vi "Meas_EIS_Spectra_Polar_v5.vi"(9 "output cluster":T1, 10 "testp":T2={"Start F"=1.0, "Stop F"=10000.0, "# Steps"=50, "Init Z Guess"=1.0, "Device #"=0, "Vdrive (V)"=0.1} caption="Test Parameters" {"Vdrive (V)" min=0.0001 max=10; "Device #" min=0 max=10 step=1; "Init Z Guess" format="%_5f"; "# Steps" min=1 max=1800 step=1; "Stop F" min=0.0010000000474974513 max=2000000.0 step=0.001 format="%#_3f"; "Start F" min=0.0010000000474974513 max=2000000.0 step=0.001 format="%#_3f"}, 11 "Output file refnum":refnum<file>) -> ()   [LabVIEW 2018]
uses:
  AC States cntrl.ctl
panel:
  out "Init Z Guess":sgl
  in  "Tab Control":enum32{"Outputs", "TakeData"}(tab)
  out "XY Graph":cluster{sgl, sgl}[](graph)
  out "IERange":i32
  out "IchRange":i32
  out "VchRange":i32
  out "Index no.":i32=1
  out "Zphz":dbl
  out "Zmod":dbl
  out "Zfreq":dbl
  in  "Control Mode":i32(ring)=1 items=["GstatMode", "PstatMode", "ZRAMode", "FRAMode"]
  out "Data Available":bool
  out "Status":enum16{"Ok", "Retry", "Error"}(ring)
  out "NumPoints":i32
  in  "Freqin":sgl=1000.0 format="%#_3g"
  out "event callback refnum":refnum<k27>
  out "Section":string
  out "ReadZ":refnum<k7>
  out "Pstat":refnum<k7>
  out "Device List":refnum<k7>
  out "Data Acquisition Complete":bool
  in  "GAMRYCOMLib.IGamryReadZ":refnum<k7>
  in  "GAMRYCOMLib.IGamryPstat":refnum<k7>
  in  "GAMRYCOMLib.IGamryDeviceList":refnum<k7>
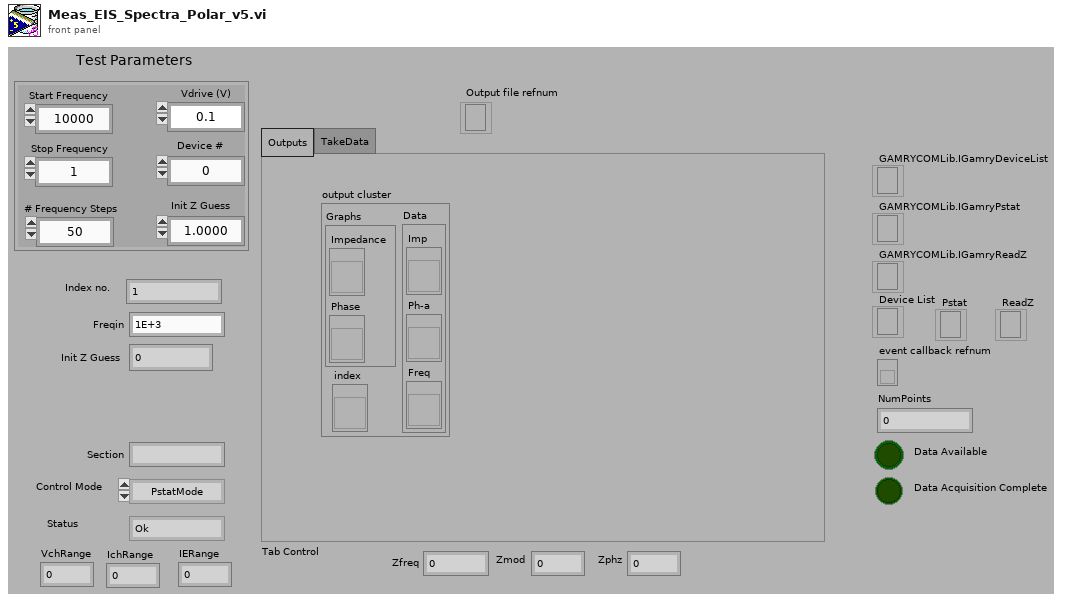
[diagram p1: front panel]
types:
  T1 = cluster{"Data":cluster{"Imp":refnum<vi>, "Ph-a":refnum<vi>, "Freq":refnum<vi>}, "Graphs":cluster{"Impedance":refnum<vi>, "Phase":refnum<vi>}, "index":refnum<vi>}
  T2 = cluster{"Start F":dbl, "Stop F":dbl, "# Steps":u32, "Init Z Guess":sgl, "Device #":i16, "Vdrive (V)":sgl}
  T3 = typedef "AC States cntrl.ctl" = enum16{"Initialize Variables", "Initialize Pstat", "Initialize Dtaq", "Settings", "Frequency calc", "Set Cycle Limits", "Take Data", "Read Z Measure", "Cleanup", "Stop"}
  T4 = cluster{"Imp":refnum<vi>, "Ph-a":refnum<vi>, "Freq":refnum<vi>}
  T5 = cluster{"Impedance":refnum<vi>, "Phase":refnum<vi>}
  T6 = cluster{"Data Acquisition Complete":refnum<vi>, "Status":refnum<vi>}
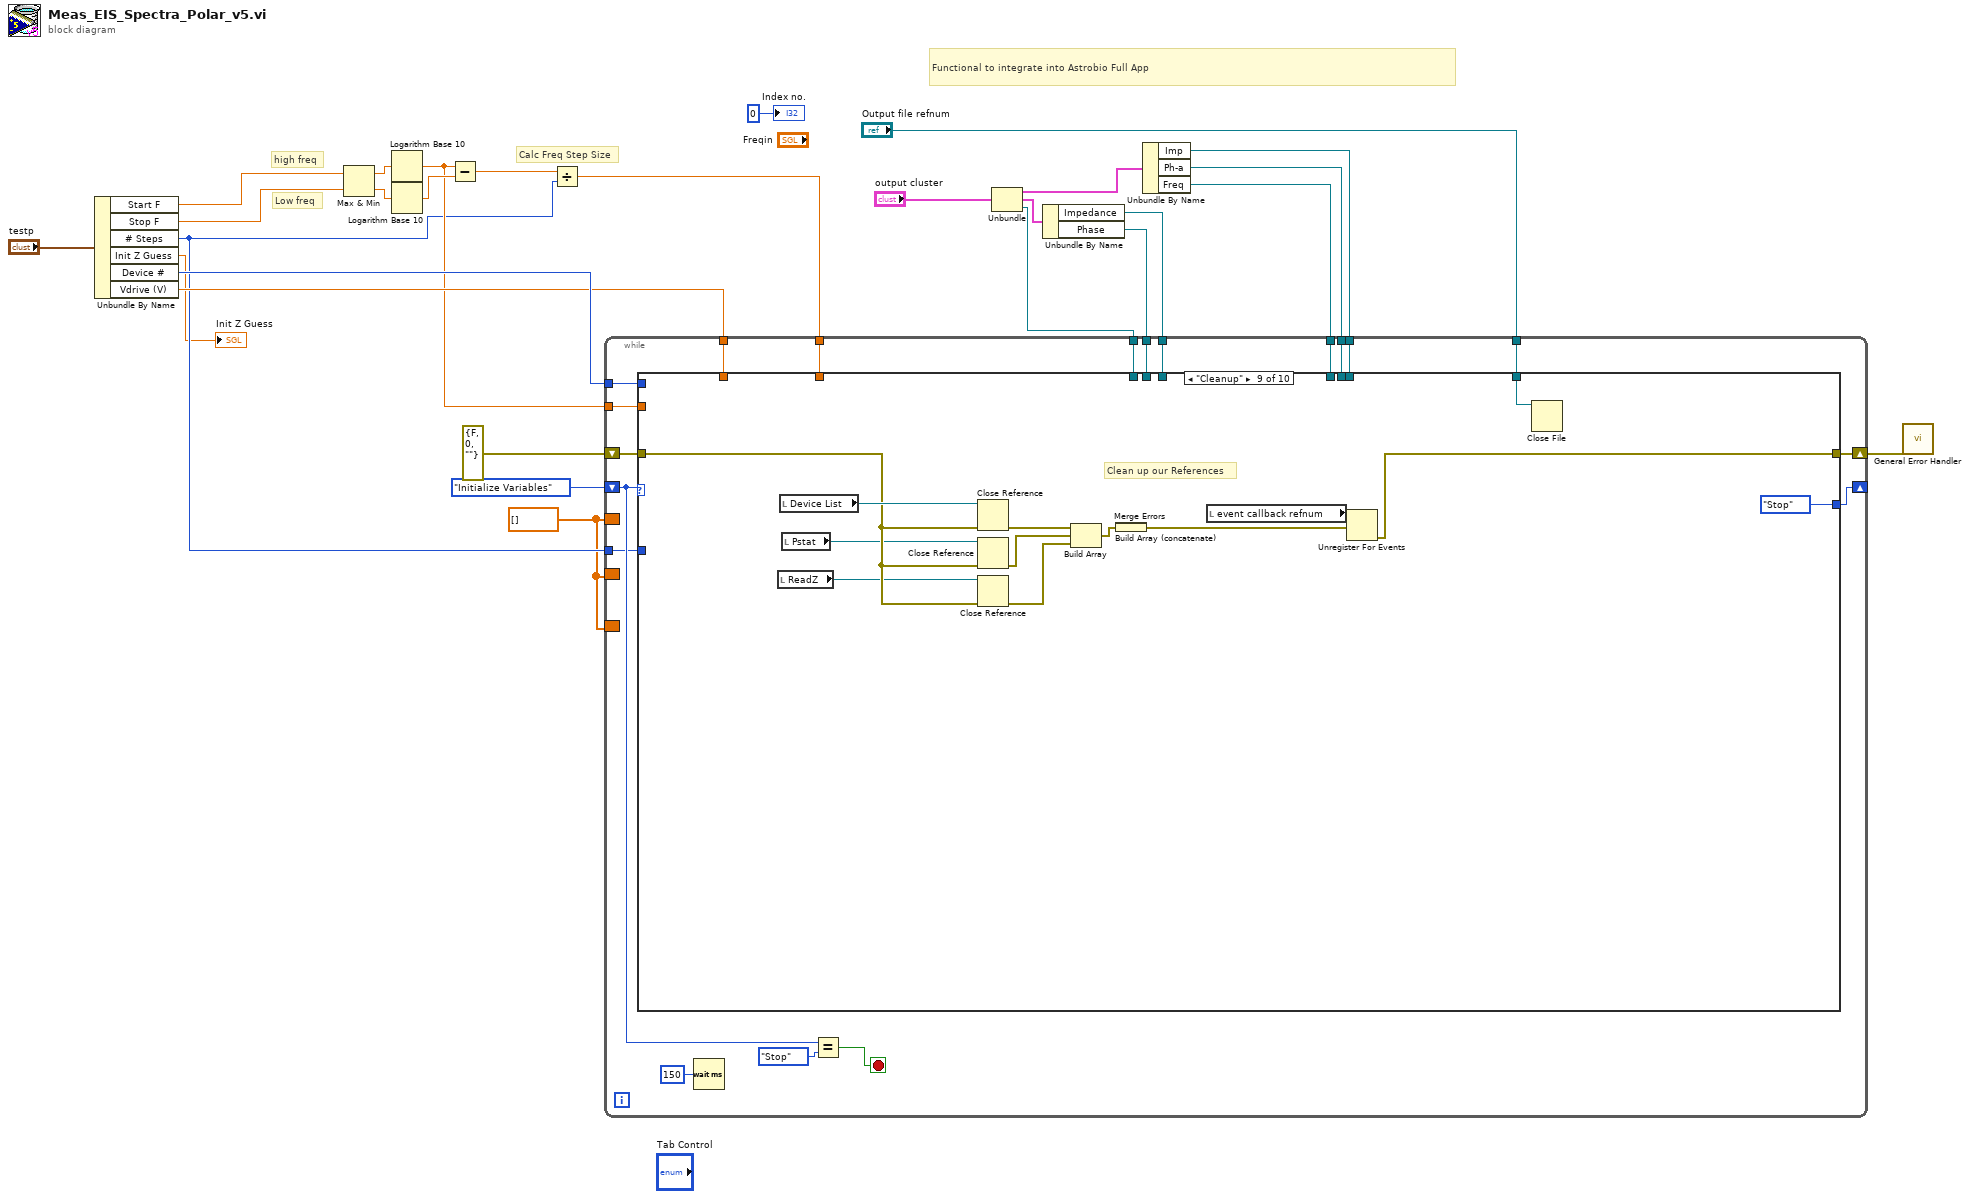
[diagram p0: block diagram]
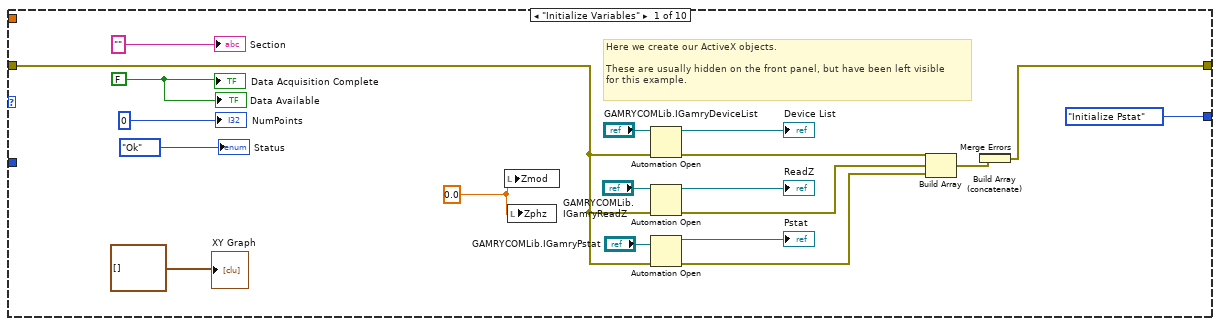
[diagram p2: hidden frame]
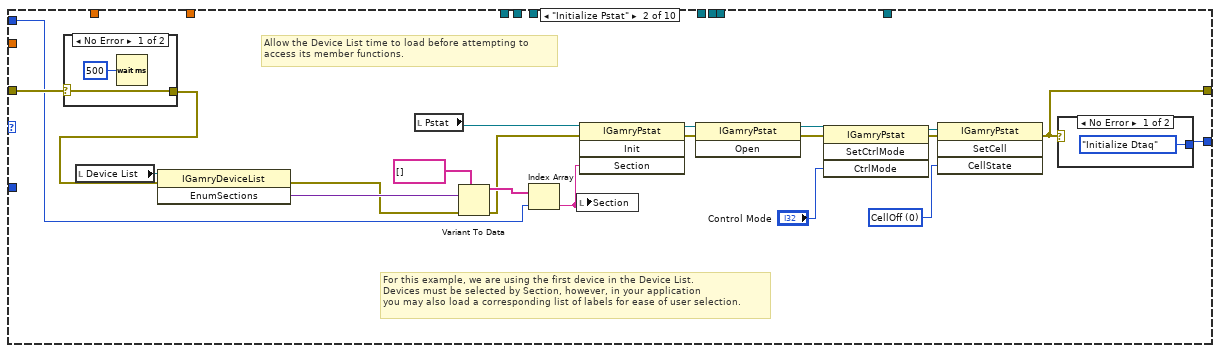
[diagram p3: hidden frame]
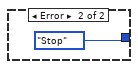
[diagram p5: hidden frame]
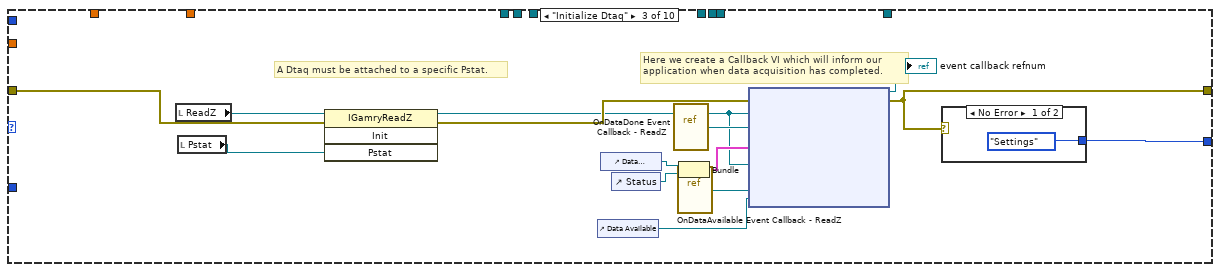
[diagram p6: hidden frame]
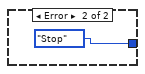
[diagram p7: hidden frame]
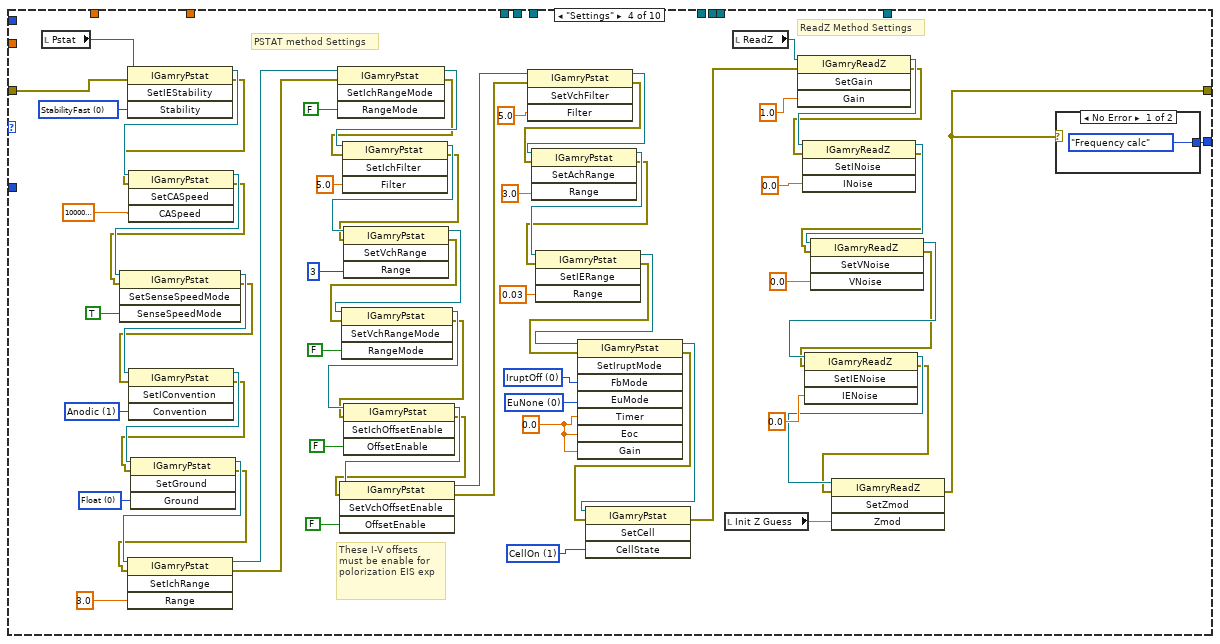
[diagram p8: hidden frame]
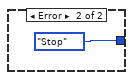
[diagram p9: hidden frame]
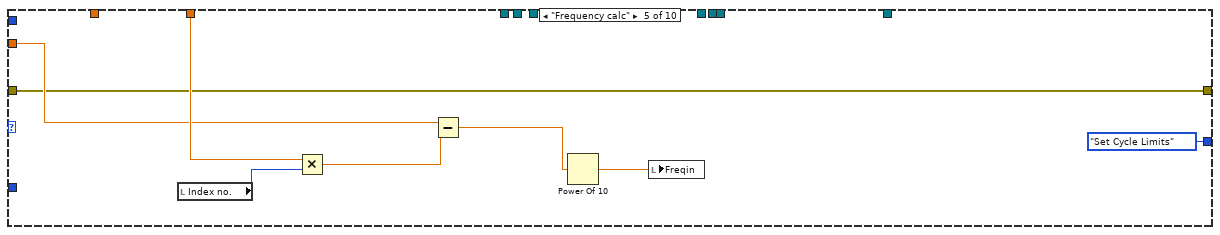
[diagram p10: hidden frame]
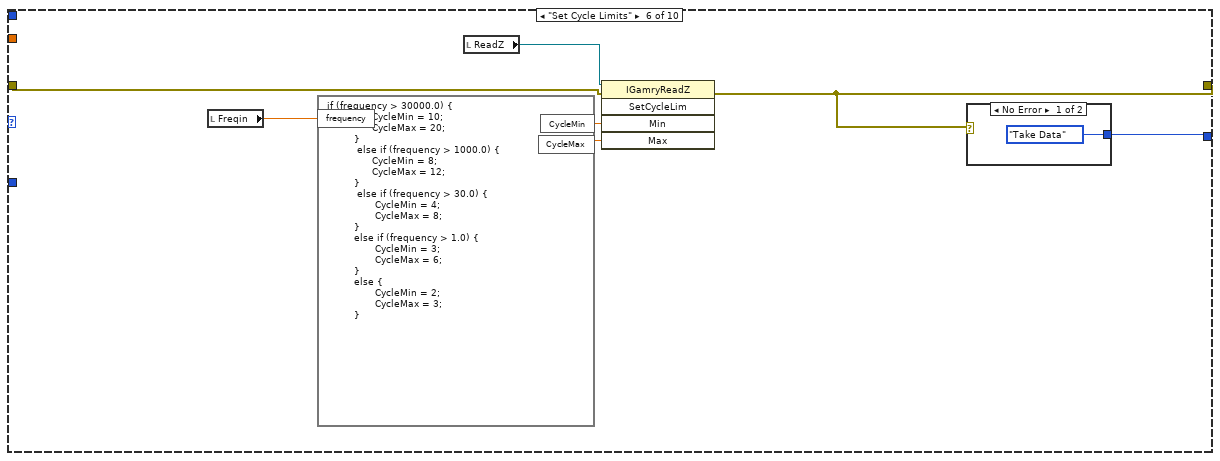
[diagram p11: hidden frame]
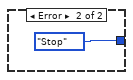
[diagram p12: hidden frame]
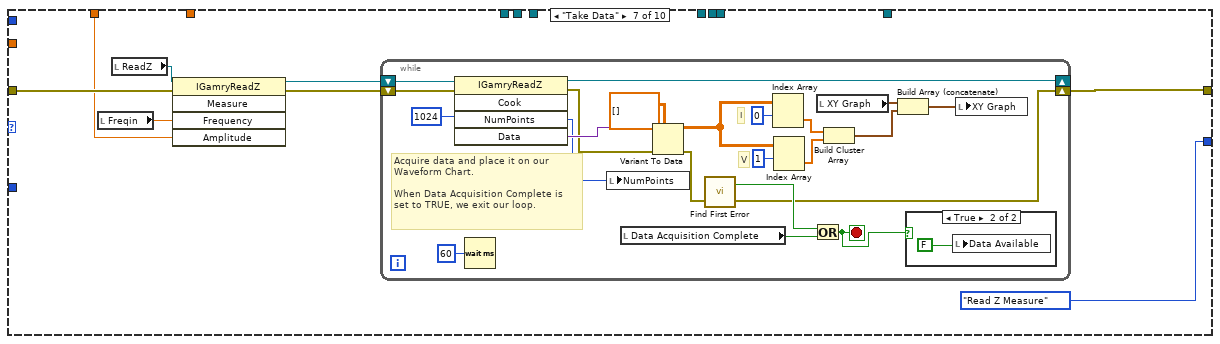
[diagram p13: hidden frame]
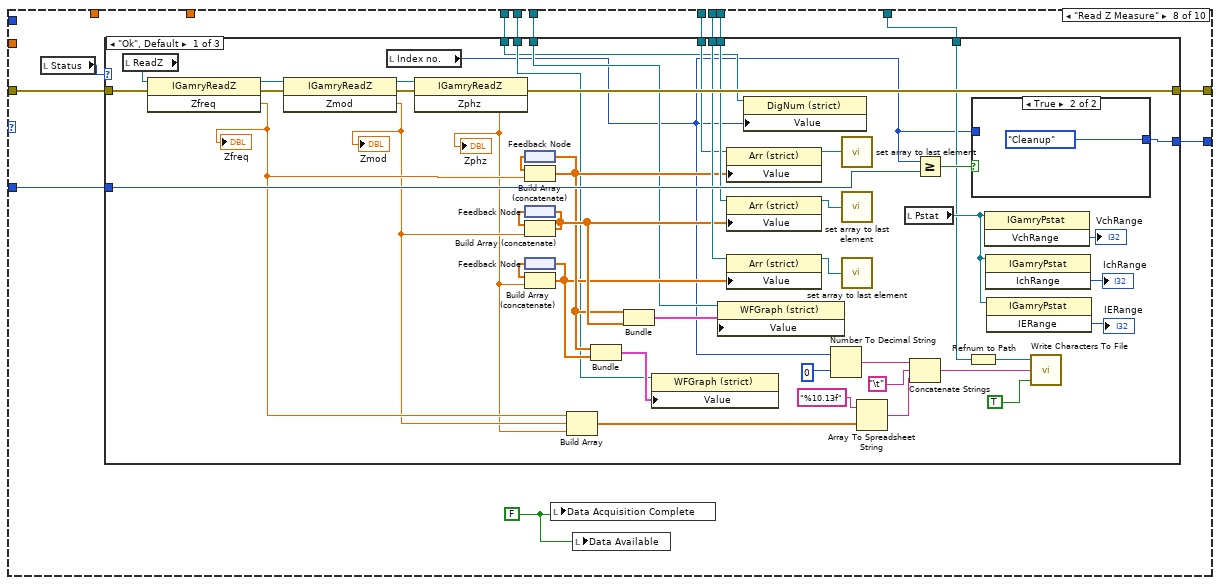
[diagram p15: hidden frame]
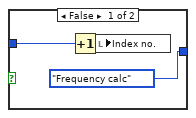
[diagram p16: hidden frame]
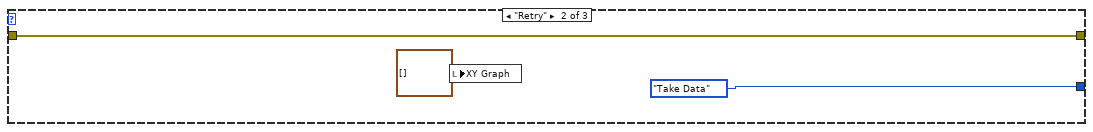
[diagram p17: hidden frame]
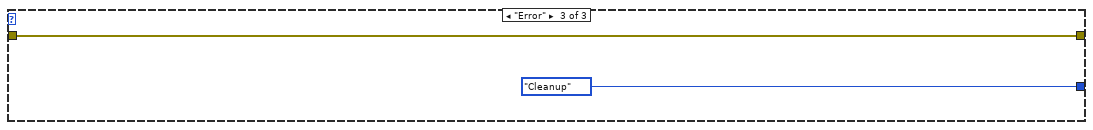
[diagram p18: hidden frame]
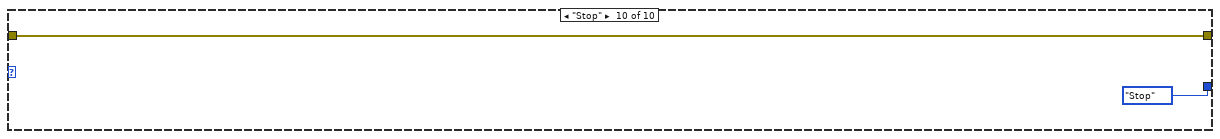
[diagram p19: hidden frame]
diagram:
  w2 = dbl[] []
  # "Functional to integrate into Astrobio Full App"
  # "Calc Freq Step Size"
  # "Low freq"
  # "high freq"
  n1 = Unbundle By Name("testp") -> ("Start F"=w18:dbl, "Stop F"=w17:dbl, "# Steps"=w13:u32, "Init Z Guess"=→"Init Z Guess":sgl, "Device #"=w24:i16, "Vdrive (V)"=w23:sgl)
  n2 = Max & Min(x=w18, y=w17) -> (max(x,y)=w21:dbl, min(x,y)=w22:dbl)
  n3 = Logarithm Base 10(1:w21) -> (0:w15:dbl)
  n4 = Logarithm Base 10(1:w22) -> (0:w19:dbl)
  n5 = Subtract(x=w15, y=w19) -> (x-y=w20:dbl)
  n6 = Divide(x=w20, y=w13) -> (x/y=w14:dbl)
  n7 = Unbundle("output cluster") -> ("Data"=w9:T4, "Graphs"=w5:T5, "index"=w1:refnum<vi>)
  n8 = Unbundle By Name(w5) -> ("Impedance"=w4:refnum<vi>, "Phase"=w3:refnum<vi>)
  n9 = Unbundle By Name(w9) -> ("Imp"=w8:refnum<vi>, "Ph-a"=w7:refnum<vi>, "Freq"=w6:refnum<vi>)
  n10 = while {
    shift-right: [w44] -> _
    shift-left: AC_States_cntrl."Initialize Variables" ("DC Demo States") -> [w45]
    shift-right: [w42] -> w27
    shift-left: errorcluster {"status"=FALSE, "code"=0, "source"=""} ("error in (no error)") -> [w43]
    tunnel: w23 -> [w40]
    tunnel: w24 -> [w39]
    tunnel: w13 -> [w38]
    tunnel: w15 -> [w37]
    tunnel: w14 -> [w36]
    tunnel: "Output file refnum" -> [w35]
    border: w2 -> [_]
    border: w2 -> [_]
    border: w2 -> [_]
    tunnel: w8 -> [w34]
    tunnel: w7 -> [w33]
    tunnel: w6 -> [w32]
    tunnel: w4 -> [w31]
    tunnel: w3 -> [w30]
    tunnel: w1 -> [w29]
    stop <- w46 stop-if-true
    n11 = case shown="\"Cleanup\"" w45 {
      tunnel: [AC_States_cntrl."Initialize Pstat" ("DC Demo States") w84 w106 w178 AC_States_cntrl."Set Cycle Limits" ("DC Demo States") w196 AC_States_cntrl."Read Z Measure" ("DC Demo States") w241 AC_States_cntrl."Stop" ("DC Demo States") AC_States_cntrl."Stop" ("DC Demo States")] -> w44
      tunnel: w43 -> [w56 w75 w104 w159 w182 w195 w205 w240 w308 w311]
      tunnel: [w57 w68 w103 w177 w182 w190 w204 w239 w299 w311] -> w42
      tunnel: w40 -> [_ _ _ _ _ _ w200 _ _ _]
      tunnel: w39 -> [_ w72 _ _ _ _ _ _ _ _]
      tunnel: w38 -> [_ _ _ _ _ _ _ w238 _ _]
      tunnel: w37 -> [_ _ _ _ w187 _ _ _ _ _]
      tunnel: w36 -> [_ _ _ _ w188 _ _ _ _ _]
      tunnel: w35 -> [_ _ _ _ _ _ _ w237 w297 _]
      tunnel: w34 -> [_ _ _ _ _ _ _ w235 _ _]
      tunnel: w33 -> [_ _ _ _ _ _ _ w234 _ _]
      tunnel: w32 -> [_ _ _ _ _ _ _ w233 _ _]
      tunnel: w31 -> [_ _ _ _ _ _ _ w232 _ _]
      tunnel: w30 -> [_ _ _ _ _ _ _ w231 _ _]
      tunnel: w29 -> [_ _ _ _ _ _ _ w230 _ _]
      frame "Initialize Variables" {
        w49 = sgl 0.0 ("Zreal")
        w51 = FALSE
        # "Here we create our ActiveX objects.\n\nThese are usually hidden on the front panel, but have been left visible\nfor this example."
        n12 = local write "Zmod"(w49) -> ()
        n13 = local write "Zphz"(w49) -> ()
        n14 = Automation Open(error in (no error)=w56, Automation Refnum="GAMRYCOMLib.IGamryDeviceList") -> (Automation Refnum=→"Device List":refnum<k7>, error out=w59:errorcluster)  [unwired: 2 in]
        n15 = Automation Open(error in (no error)=w56, Automation Refnum="GAMRYCOMLib.IGamryReadZ") -> (Automation Refnum=→"ReadZ":refnum<k7>, error out=w54:errorcluster)  [unwired: 2 in]
        n16 = Automation Open(error in (no error)=w56, Automation Refnum="GAMRYCOMLib.IGamryPstat") -> (Automation Refnum=→"Pstat":refnum<k7>, error out=w55:errorcluster)  [unwired: 2 in]
        n17 = Build Array(w59, w54, w55) -> (w58:errorcluster[])
        n18 = Build Array (concatenate)(w58) -> (w50:errorcluster[])
        n19 = Merge Errors(w50) -> (w57:errorcluster)
        "Data Acquisition Complete" <- w51
        "Section" <- "" ("Section")
        "NumPoints" <- 0 ("NumPoints")
        "Data Available" <- w51
        "XY Graph" <- cluster{sgl, sgl}[] [] ("appended array")
        "Status" <- enum16{"Ok", "Retry", "Error"}."Ok" ("Status")
      }
      frame "Initialize Pstat" {
        w71 = 0 items=["CellOff", "CellOn"] ("CellState")
        # "For this example, we are using the first device in the Device List.\nDevices must be selected by Section, however, in your application\nyou may also load a corresponding list of labels for ease of user selection."
        # "Allow the Device List time to load before attempting to \naccess its member functions."
        n20 = case shown="No Error" w75 {
          selector: w75 -> [w89 w91]
          tunnel: [w89 w91] -> w74
          frame No Error {
            n21 = Wait (ms)(milliseconds to wait=u32 500) -> ()  [unwired: 1 out]
          }
          frame Error {
          }
        }
        n22 = local read "Device List"() -> (w79:refnum<k7>)
        n23 = invoke class="IGamryDeviceList" method="EnumSections"(reference=w79, error in=w74) -> (error out=w77:errorcluster, "EnumSections"=w78:variant)  [unwired: 1 in, 1 out]
        n24 = local read "Pstat"() -> (w81:refnum<k7>)
        n25 = Variant To Data(error in=w77, type=string[] [], Variant=w78) -> (data=w83:string[], error out=w76:errorcluster)
        n26 = Index Array(array=w83, index=w72) -> (element=w80:string)
        n27 = local write "Section"(w80) -> ()
        n28 = invoke class="IGamryPstat" method="Init"(reference=w81, error in=w76, "Section"=w80) -> (reference out=w88:refnum<k7>, error out=w87:errorcluster)  [unwired: 1 in, 2 out]
        n29 = invoke class="IGamryPstat" method="Open"(reference=w88, error in=w87) -> (reference out=w85:refnum<k7>, error out=w86:errorcluster)  [unwired: 1 in, 1 out]
        n30 = invoke class="IGamryPstat" method="SetCtrlMode"(reference=w85, error in=w86, "CtrlMode"="Control Mode") -> (reference out=w70:refnum<k7>, error out=w69:errorcluster)  [unwired: 1 in, 2 out]
        n31 = invoke class="IGamryPstat" method="SetCell"(reference=w70, error in=w69, "CellState"=w71) -> (error out=w68:errorcluster)  [unwired: 1 in, 3 out]
        n32 = case shown="No Error" w68 {
          tunnel: [AC_States_cntrl."Initialize Dtaq" ("DC Demo States") AC_States_cntrl."Stop" ("DC Demo States")] -> w84
          frame No Error {
          }
          frame Error {
          }
        }
      }
      frame "Initialize Dtaq" {
        # "A Dtaq must be attached to a specific Pstat."
        # "Here we create a Callback VI which will inform our\napplication when data acquisition has completed."
        n33 = local read "ReadZ"() -> (w105:refnum<k7>)
        n34 = local read "Pstat"() -> (w107:refnum<k7>)
        n35 = invoke class="IGamryReadZ" method="Init"(reference=w105, error in=w104, "Pstat"=w107) -> (reference out=w95:refnum<k7>, error out=w101:errorcluster)  [unwired: 1 in, 2 out]
        n36 = control-ref of="Data Available"() -> (w96:refnum<vi>)
        n37 = control-ref of="Data Acquisition Complete"() -> (w100:refnum<vi>)
        n38 = control-ref of="Status"() -> (w99:refnum<vi>)
        n39 = vi-ref "OnDataDone Event Callback - ReadZ.vi"() -> ("vi reference"=w97:refnum<vi>)
        n40 = vi-ref "OnDataAvailable Event Callback - ReadZ.vi"() -> ("vi reference"=w94:refnum<vi>)
        n41 = Bundle("Data Acquisition Complete"=w100, "Status"=w99) -> (w98:T6)  [unwired: 1 in]
        n42 = node(w101, w95, w97, w98, w95, w94, w96) -> (→"event callback refnum":refnum<k27>, w103:errorcluster)  [unwired: 1 in]
        n43 = case shown="No Error" w103 {
          tunnel: [AC_States_cntrl."Settings" ("DC Demo States") AC_States_cntrl."Stop" ("DC Demo States")] -> w106
          frame No Error {
          }
          frame Error {
          }
        }
      }
      frame "Settings" {
        w113 = sgl 0.0 ("Timer")
        w114 = 0 items=["EuNone", "EuExtrap", "EuAverage"] ("EuMode")
        w115 = 0 items=["IruptOff", "IruptNorm", "IruptClfg"] ("FbMode")
        w148 = 0 items=["Float", "Earth"] ("Ground")
        w151 = 1 items=["Cathodic", "Anodic"] ("Convention")
        w158 = 0 items=["StabilityFast", "StabilityMedFast", "StabilityNorm", "StabilitySlow"] ("Stability")
        w179 = 1 items=["CellOff", "CellOn"] ("CellState")
        # "ReadZ Method Settings"
        # "These I-V offsets must be enable for polorization EIS exp"
        # "PSTAT method Settings"
        n44 = local read "Pstat"() -> (w160:refnum<k7>)
        n45 = invoke class="IGamryPstat" method="SetIEStability"(reference=w160, error in=w159, "Stability"=w158) -> (reference out=w157:refnum<k7>, error out=w156:errorcluster)  [unwired: 1 in, 2 out]
        n46 = invoke class="IGamryPstat" method="SetCASpeed"(reference=w157, error in=w156, "CASpeed"=1000000.0) -> (reference out=w153:refnum<k7>, error out=w152:errorcluster)  [unwired: 1 in, 2 out]
        n47 = invoke class="IGamryPstat" method="SetSenseSpeedMode"(reference=w153, error in=w152, "SenseSpeedMode"=TRUE) -> (reference out=w150:refnum<k7>, error out=w149:errorcluster)  [unwired: 1 in, 2 out]
        n48 = invoke class="IGamryPstat" method="SetIConvention"(reference=w150, error in=w149, "Convention"=w151) -> (reference out=w147:refnum<k7>, error out=w146:errorcluster)  [unwired: 1 in, 2 out]
        n49 = invoke class="IGamryPstat" method="SetGround"(reference=w147, error in=w146, "Ground"=w148) -> (reference out=w144:refnum<k7>, error out=w143:errorcluster)  [unwired: 1 in, 2 out]
        n50 = invoke class="IGamryPstat" method="SetIchRange"(reference=w144, error in=w143, "Range"=3.0) -> (reference out=w142:refnum<k7>, error out=w141:errorcluster)  [unwired: 1 in, 2 out]
        n51 = invoke class="IGamryPstat" method="SetIchRangeMode"(reference=w142, error in=w141, "RangeMode"=FALSE) -> (reference out=w138:refnum<k7>, error out=w137:errorcluster)  [unwired: 1 in, 2 out]
        n52 = invoke class="IGamryPstat" method="SetIchFilter"(reference=w138, error in=w137, "Filter"=5.0) -> (reference out=w136:refnum<k7>, error out=w135:errorcluster)  [unwired: 1 in, 2 out]
        n53 = invoke class="IGamryPstat" method="SetVchRange"(reference=w136, error in=w135, "Range"=3) -> (reference out=w133:refnum<k7>, error out=w132:errorcluster)  [unwired: 1 in, 2 out]
        n54 = invoke class="IGamryPstat" method="SetVchRangeMode"(reference=w133, error in=w132, "RangeMode"=FALSE) -> (reference out=w131:refnum<k7>, error out=w130:errorcluster)  [unwired: 1 in, 2 out]
        n55 = invoke class="IGamryPstat" method="SetIchOffsetEnable"(reference=w131, error in=w130, "OffsetEnable"=FALSE) -> (reference out=w127:refnum<k7>, error out=w126:errorcluster)  [unwired: 1 in, 2 out]
        n56 = invoke class="IGamryPstat" method="SetVchOffsetEnable"(reference=w127, error in=w126, "OffsetEnable"=FALSE) -> (reference out=w125:refnum<k7>, error out=w124:errorcluster)  [unwired: 1 in, 2 out]
        n57 = invoke class="IGamryPstat" method="SetVchFilter"(reference=w125, error in=w124, "Filter"=5.0) -> (reference out=w121:refnum<k7>, error out=w120:errorcluster)  [unwired: 1 in, 2 out]
        n58 = invoke class="IGamryPstat" method="SetAchRange"(reference=w121, error in=w120, "Range"=3.0) -> (reference out=w119:refnum<k7>, error out=w118:errorcluster)  [unwired: 1 in, 2 out]
        n59 = invoke class="IGamryPstat" method="SetIERange"(reference=w119, error in=w118, "Range"=0.03) -> (reference out=w117:refnum<k7>, error out=w116:errorcluster)  [unwired: 1 in, 2 out]
        n60 = invoke class="IGamryPstat" method="SetIruptMode"(reference=w117, error in=w116, "FbMode"=w115, "EuMode"=w114, "Timer"=w113, "Eoc"=w113, "Gain"=w113) -> (reference out=w112:refnum<k7>, error out=w111:errorcluster)  [unwired: 1 in, 6 out]
        n61 = invoke class="IGamryPstat" method="SetCell"(reference=w112, error in=w111, "CellState"=w179) -> (error out=w174:errorcluster)  [unwired: 1 in, 3 out]
        n62 = local read "Init Z Guess"() -> (w110:sgl)
        n63 = local read "ReadZ"() -> (w175:refnum<k7>)
        n64 = invoke class="IGamryReadZ" method="SetGain"(reference=w175, error in=w174, "Gain"=sgl 1.0 ("Zmod")) -> (reference out=w172:refnum<k7>, error out=w171:errorcluster)  [unwired: 1 in, 2 out]
        n65 = invoke class="IGamryReadZ" method="SetINoise"(reference=w172, error in=w171, "INoise"=sgl 0.0 ("Zmod")) -> (reference out=w169:refnum<k7>, error out=w168:errorcluster)  [unwired: 1 in, 2 out]
        n66 = invoke class="IGamryReadZ" method="SetVNoise"(reference=w169, error in=w168, "VNoise"=sgl 0.0 ("Zmod")) -> (reference out=w166:refnum<k7>, error out=w165:errorcluster)  [unwired: 1 in, 2 out]
        n67 = invoke class="IGamryReadZ" method="SetIENoise"(reference=w166, error in=w165, "IENoise"=sgl 0.0 ("Zmod")) -> (reference out=w164:refnum<k7>, error out=w163:errorcluster)  [unwired: 1 in, 2 out]
        n68 = invoke class="IGamryReadZ" method="SetZmod"(reference=w164, error in=w163, "Zmod"=w110) -> (error out=w177:errorcluster)  [unwired: 1 in, 3 out]
        n69 = case shown="No Error" w177 {
          tunnel: [AC_States_cntrl."Frequency calc" ("DC Demo States") AC_States_cntrl."Stop" ("DC Demo States")] -> w178
          frame No Error {
          }
          frame Error {
          }
        }
      }
      frame "Frequency calc" {
        n70 = local read "Index no."() -> (w189:i32)
        n71 = Multiply(x=w188, y=w189) -> (x*y=w186:dbl)
        n72 = Subtract(x=w187, y=w186) -> (x-y=w185:dbl)
        n73 = Power Of 10(x=w185) -> (10^x=w184:dbl)
        n74 = local write "Freqin"(w184) -> ()
      }
      frame "Set Cycle Limits" {
        n75 = local read "Freqin"() -> (w193:sgl)
        n76 = formula code="if (frequency > 30000.0) {\n               CycleMin = 10;\n               CycleMax = 20;\n         }\n          else if (frequency > 1000.0) {\n               CycleMin = 8;\n               CycleMax = 12;\n         }\n          else if (frequency > 30.0) {\n                CycleMin = 4;\n                CycleMax = 8;\n         }\n         else if (frequency > 1.0) {\n                CycleMin = 3;\n                CycleMax = 6;\n         }\n         else {\n                CycleMin = 2;\n                CycleMax = 3;\n         }"("frequency"=w193) -> ("CycleMin"=w192:dbl, "CycleMax"=w191:dbl)
        n77 = local read "ReadZ"() -> (w194:refnum<k7>)
        n78 = invoke class="IGamryReadZ" method="SetCycleLim"(reference=w194, error in=w195, "Min"=w192, "Max"=w191) -> (error out=w190:errorcluster)  [unwired: 1 in, 4 out]
        n79 = case shown="No Error" w190 {
          tunnel: [AC_States_cntrl."Take Data" ("DC Demo States") AC_States_cntrl."Stop" ("DC Demo States")] -> w196
          frame No Error {
          }
          frame Error {
          }
        }
      }
      frame "Take Data" {
        n80 = local read "Freqin"() -> (w199:sgl)
        n81 = local read "ReadZ"() -> (w203:refnum<k7>)
        n82 = invoke class="IGamryReadZ" method="Measure"(reference=w203, error in=w205, "Frequency"=w199, "Amplitude"=w200) -> (reference out=w202:refnum<k7>, error out=w201:errorcluster)  [unwired: 1 in, 3 out]
        n83 = while {
          shift-right: [w219] -> w204
          shift-left: w201 -> [w227]
          shift-right: [w218] -> _
          shift-left: w202 -> [w228]
          stop <- w207 stop-if-true
          # "V"
          # "I"
          # "Acquire data and place it on our\nWaveform Chart.\n\nWhen Data Acquisition Complete is\nset to TRUE, we exit our loop."
          n84 = invoke class="IGamryReadZ" method="Cook"(reference=w228, error in=w227, "NumPoints"=1024) -> (reference out=w218:refnum<k7>, error out=w223:errorcluster, "NumPoints"=w213:i32, "Data"=w224:variant)  [unwired: 2 in, 1 out]
          n85 = Wait (ms)(milliseconds to wait=u32 60) -> ()  [unwired: 1 out]
          n86 = local write "NumPoints"(w213) -> ()
          n87 = local read "Data Acquisition Complete"() -> (w220:bool)
          n88 = Variant To Data(error in=w223, type=sgl[][] [], Variant=w224) -> (data=w214:sgl[][], error out=w222:errorcluster)
          n89 = call <vilib>:"Find First Error.vi"("error in (no error)"=w222) -> ("error out"=w219:errorcluster, "error?"=w221:bool)  [unwired: 3 in]
          n90 = Index Array(array=w214, index (row)=0) -> (element=w212:sgl[])  [unwired: 1 in]
          n91 = Index Array(array=w214, index (row)=1) -> (element=w211:sgl[])  [unwired: 1 in]
          n92 = Or(x=w221, y=w220) -> (x .or. y?=w207:bool)
          n93 = local read "XY Graph"() -> (w210:cluster{sgl, sgl}[])
          n94 = Build Cluster Array(w212, w211) -> (w209:cluster{sgl, sgl}[])
          n95 = Build Array (concatenate)(w210, w209) -> (w208:cluster{sgl, sgl}[])
          n96 = case shown="True" w207 {
            frame False {
            }
            frame True {
              n97 = local write "Data Available"(FALSE) -> ()
            }
          }
          n98 = local write "XY Graph"(w208) -> ()
        }
      }
      frame "Read Z Measure" {
        w236 = FALSE
        n99 = local read "Status"() -> (w242:enum16{"Ok", "Retry", "Error"})
        n100 = case shown="\"Ok\", Default" w242 {
          tunnel: [w274 AC_States_cntrl."Take Data" ("DC Demo States") AC_States_cntrl."Cleanup" ("DC Demo States")] -> w241
          tunnel: w240 -> [w284 w293 w295]
          tunnel: [w285 w293 w295] -> w239
          tunnel: w238 -> [w276 _ _]
          tunnel: w237 -> [w265 _ _]
          tunnel: w235 -> [w257 _ _]
          tunnel: w234 -> [w256 _ _]
          tunnel: w233 -> [w255 _ _]
          tunnel: w232 -> [w249 _ _]
          tunnel: w231 -> [w248 _ _]
          tunnel: w230 -> [w247 _ _]
          frame "Ok", Default {
            n101 = local read "ReadZ"() -> (w281:refnum<k7>)
            n102 = invoke class="IGamryReadZ" method="Zfreq"(reference=w281, error in=w284) -> (reference out=w282:refnum<k7>, error out=w283:errorcluster, "Zfreq"=w261:sgl)  [unwired: 1 in]
            "Zfreq" <- w261
            n103 = invoke class="IGamryReadZ" method="Zmod"(reference=w282, error in=w283) -> (reference out=w286:refnum<k7>, error out=w287:errorcluster, "Zmod"=w260:sgl)  [unwired: 1 in]
            "Zmod" <- w260
            n104 = local read "Index no."() -> (w246:i32)
            n105 = invoke class="IGamryReadZ" method="Zphz"(reference=w286, error in=w287) -> (error out=w285:errorcluster, "Zphz"=w258:sgl)  [unwired: 1 in, 1 out]
            "Zphz" <- w258
            n106 = feedback #1() -> (w244:dbl[])
            n107 = Build Array (concatenate)(w244, w261) -> (w252:dbl[])
            n108 = feedback-in #1(w252) -> ()
            n109 = feedback #2() -> (w259:dbl[])
            n110 = Build Array (concatenate)(w259, w260) -> (w253:dbl[])
            n111 = feedback-in #2(w253) -> ()
            n112 = feedback #3() -> (w245:dbl[])
            n113 = Build Array (concatenate)(w245, w258) -> (w251:dbl[])
            n114 = feedback-in #3(w251) -> ()
            n115 = Build Array(w261, w260, w258) -> (w271:sgl[])
            n116 = Bundle(w252, w251) -> (w250:cluster{dbl[], dbl[]})  [unwired: 1 in]
            n117 = Bundle(w252, w253) -> (w254:cluster{dbl[], dbl[]})  [unwired: 1 in]
            n118 = property class="WFGraph (strict)"(reference=w248, "Value"=w250) -> ()  [unwired: 1 in, 2 out]
            n119 = property class="WFGraph (strict)"(reference=w249, "Value"=w254) -> ()  [unwired: 1 in, 2 out]
            n120 = property class="Arr (strict)"(reference=w255, "Value"=w252) -> (reference out=w264:refnum<vi>)  [unwired: 1 in, 1 out]
            n121 = property class="Arr (strict)"(reference=w257, "Value"=w253) -> (reference out=w263:refnum<vi>)  [unwired: 1 in, 1 out]
            n122 = property class="Arr (strict)"(reference=w256, "Value"=w251) -> (reference out=w262:refnum<vi>)  [unwired: 1 in, 1 out]
            n123 = property class="DigNum (strict)"(reference=w247, "Value"=w246) -> ()  [unwired: 1 in, 2 out]
            n124 = Number To Decimal String(number=w246, width (-)=i16 0) -> (decimal integer string=w268:string)
            n125 = call "set array to last element.vi"("Arr Refnum"=w264) -> ()
            n126 = call "set array to last element.vi"("Arr Refnum"=w263) -> ()
            n127 = call "set array to last element.vi"("Arr Refnum"=w262) -> ()
            n128 = Array To Spreadsheet String(array=w271, 3:"%10.13f") -> (spreadsheet string=w267:string)  [unwired: 1 in]
            n129 = local read "Pstat"() -> (w280:refnum<k7>)
            n130 = Concatenate Strings(w268, "\t", w267) -> (w266:string)
            n131 = Greater Or Equal?(x=w246, y=w276) -> (x >= y?=w275:bool)
            n132 = Refnum to Path(1:w265) -> (0:w243:path)
            n133 = case shown="True" w275 {
              tunnel: [AC_States_cntrl."Frequency calc" ("DC Demo States") AC_States_cntrl."Cleanup" ("DC Demo States")] -> w274
              tunnel: w246 -> [w288 _]
              frame False {
                n134 = Increment(x=w288) -> (x+1=w289:i32)
                n135 = local write "Index no."(w289) -> ()
              }
              frame True {
              }
            }
            n136 = invoke class="IGamryPstat" method="VchRange"(reference=w280) -> ("VchRange"=→"VchRange":i32)  [unwired: 2 in, 2 out]
            n137 = invoke class="IGamryPstat" method="IchRange"(reference=w280) -> ("IchRange"=→"IchRange":i32)  [unwired: 2 in, 2 out]
            n138 = invoke class="IGamryPstat" method="IERange"(reference=w280) -> ("IERange"=→"IERange":i32)  [unwired: 2 in, 2 out]
            n139 = call <vilib>:"Write Characters To File.vi"("append to file? (new file:F)"=TRUE, "character string"=w266, "file path (dialog if empty)"=w243) -> ()  [unwired: 2 in, 1 out]
          }
          frame "Retry" {
            n140 = local write "XY Graph"(cluster{sgl, sgl}[] [] ("appended array")) -> ()
          }
          frame "Error" {
          }
        }
        n141 = local write "Data Acquisition Complete"(w236) -> ()
        n142 = local write "Data Available"(w236) -> ()
      }
      frame "Cleanup" {
        # "Clean up our References"
        n143 = local read "ReadZ"() -> (w306:refnum<k7>)
        n144 = local read "Device List"() -> (w309:refnum<k7>)
        n145 = local read "Pstat"() -> (w307:refnum<k7>)
        n146 = Close Reference(reference=w309, error in (no error)=w308) -> (error out=w305:errorcluster)
        n147 = Close Reference(reference=w307, error in (no error)=w308) -> (error out=w304:errorcluster)
        n148 = Close Reference(reference=w306, error in (no error)=w308) -> (error out=w303:errorcluster)
        n149 = Build Array(w305, w304, w303) -> (w302:errorcluster[])
        n150 = Build Array (concatenate)(w302) -> (w298:errorcluster[])
        n151 = Merge Errors(w298) -> (w300:errorcluster)
        n152 = local read "event callback refnum"() -> (w301:refnum<k27>)
        n153 = Unregister For Events(event registration refnum=w301, error in=w300) -> (error out=w299:errorcluster)
        n154 = Close File(refnum=w297) -> ()  [unwired: 1 in, 2 out]
      }
      frame "Stop" {
      }
    }
    n155 = Wait (ms)(milliseconds to wait=u32 150) -> ()  [unwired: 1 out]
    n156 = Equal?(x=w45, y=AC_States_cntrl."Stop" ("DC Demo States")) -> (x = y?=w46:bool)
  }
  n157 = call <vilib>:"General Error Handler.vi"("error in (no error)"=w27) -> ()  [unwired: 10 in, 5 out]
  "Index no." <- 0 ("Index no.")
